vi "DCIMG_readmetadata_multiple files.vi"(0 "Volume number":dbl, 5 "Input File Path":path, 7 "Input File Name":string, 9 "Output Path":path, 11 "error in (no error)":errorcluster) -> (6 "Metadata":string, 8 "Total":i32, 13 "Error Out":errorcluster)   [LabVIEW 2016]
panel:
  # "This is an example of how to read the images\nwithin a DCIMG file and write them to TIFF files."
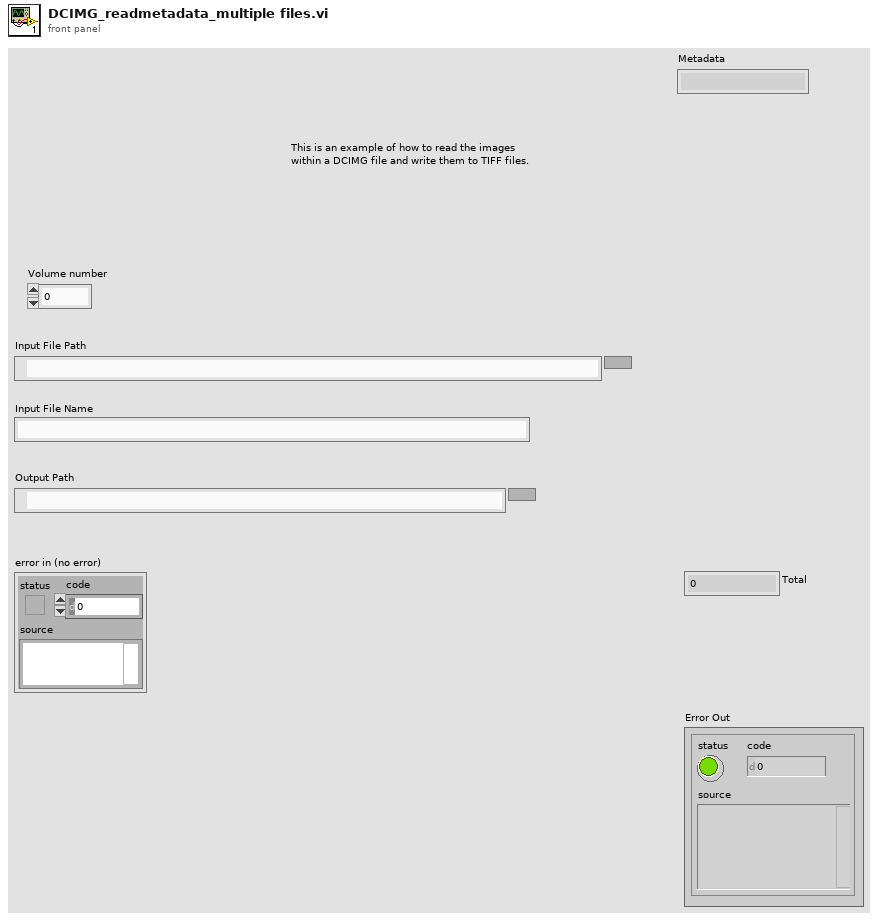
[diagram p1: front panel]
types:
  T1 = cluster{"Rows Per Strip":i32, "Photometric":i32, "Compression Type":i32}
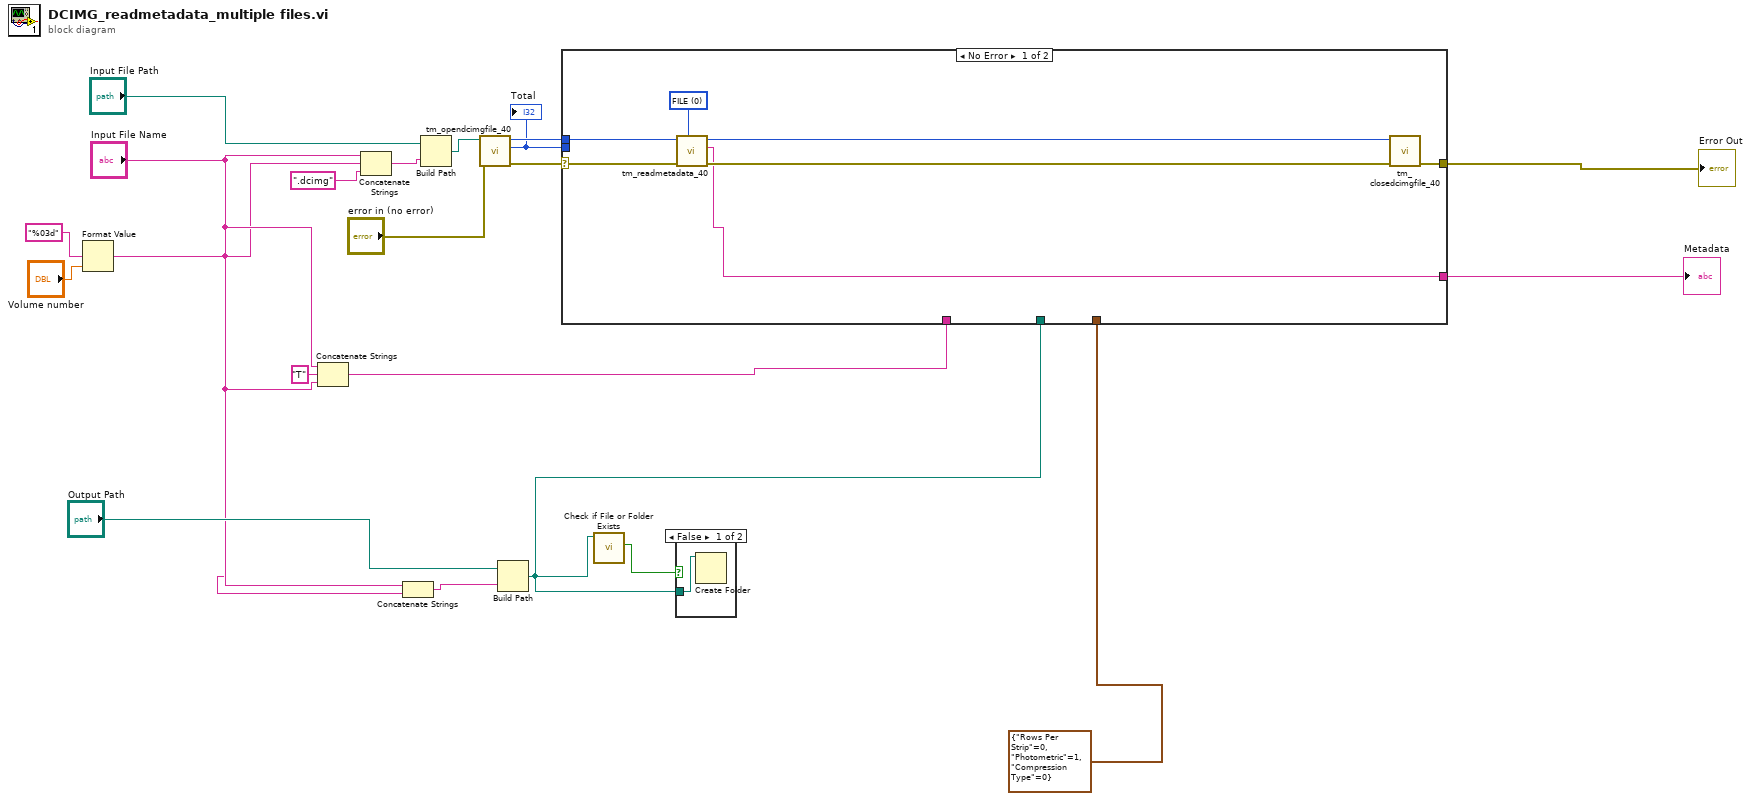
[diagram p0: block diagram]
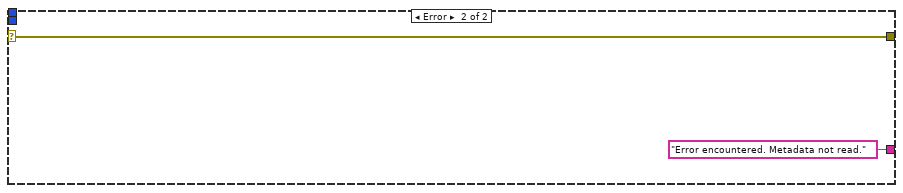
[diagram p3: hidden frame]
diagram:
  n1 = Format Value(format string="%03d", value (0)="Volume number") -> (output string=w15:string)  [unwired: 1 in]
  n2 = Concatenate Strings("Input File Name", "T" ("string"), w15) -> (w2:string)
  n3 = Concatenate Strings("Input File Name", w15, ".dcimg" ("string")) -> (w3:string)
  n4 = Concatenate Strings("Input File Name", w15) -> (w6:string)
  n5 = Build Path(base path="Input File Path", name or relative path=w3) -> (appended path=w5:path)
  n6 = call <userlib>:"tm_opendcimgfile_40.vi"("error in (no error)"="error in (no error)", "Path"=w5) -> ("error out"=w12:errorcluster, "Total Frames"=w10:i32, "File Handle"=w11:u32)  [unwired: 7 in]
  "Total" <- w10
  n7 = Build Path(base path="Output Path", name or relative path=w6) -> (appended path=w7:path)
  n8 = case shown="No Error" w12 {
    selector: w12 -> [w26 w30]
    tunnel: w11 -> [w27 _]
    tunnel: [w28 w30] -> w21
    tunnel: w10 -> [_ _]
    tunnel: w7 -> [_ _]
    tunnel: w2 -> [_ _]
    tunnel: T1 {"Rows Per Strip"=0, "Photometric"=1, "Compression Type"=0} ("TIFF Options") -> [_ _]
    tunnel: [w22 "Error encountered. Metadata not read." ("Metadata")] -> w13
    frame No Error {
      w25 = 0 items=["FILE"=0, "FRAME"=2] ("Type")
      n9 = call <userlib>:"tm_readmetadata_40.vi"("Type"=w25, "error in (no error)"=w26, "File Handle"=w27) -> ("error out"=w23:errorcluster, "Metadata"=w22:string, "File Handle"=w24:u32)  [unwired: 6 in]
      n10 = call <userlib>:"tm_closedcimgfile_40.vi"("error in (no error)"=w23, "File Handle"=w24) -> ("error out"=w28:errorcluster)  [unwired: 9 in]
    }
    frame Error {
    }
  }
  "Error Out" <- w21
  "Metadata" <- w13
  n11 = call <vilib>:"Check if File or Folder Exists.vi"("path"=w7) -> ("file or folder exists?"=w8:bool)  [unwired: 8 in, 2 out]
  n12 = case shown="False" w8 {
    tunnel: w7 -> [w31 _]
    frame False {
      n13 = Create Folder(path (use dialog)=w31) -> ()  [unwired: 2 in, 3 out]
    }
    frame True {
    }
  }
